vi "DeleteLongFolderStuctureFromSaveAsPrevious.vi"(8 "error in (no error)":errorcluster, 11 "Path":path) -> ()   [LabVIEW 2016]
panel:
  out "appended path":path
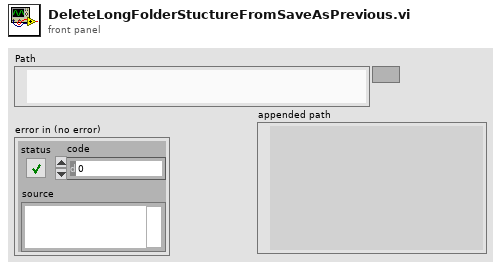
[diagram p1: front panel]
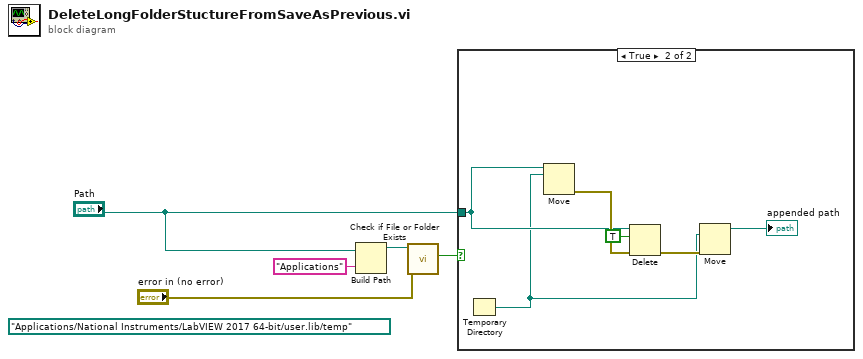
[diagram p0: block diagram]
diagram:
  (unwired) path "Applications/National Instruments/LabVIEW 2017 64-bit/user.lib/temp" ("Path")
  n1 = Build Path(base path="Path", name or relative path="Applications") -> (appended path=w1:path)
  n2 = call <vilib>:"Check if File or Folder Exists.vi"("error in (no error)"="error in (no error)", "path"=w1) -> ("file or folder exists?"=w3:bool)  [unwired: 7 in, 2 out]
  n3 = case shown="True" w3 {
    tunnel: "Path" -> [_ w7]
    frame False {
    }
    frame True {
      n4 = Temporary Directory() -> (w6:path)
      n5 = Move(source path=w7, 10:w6) -> (error out=w11:errorcluster)  [unwired: 3 in, 2 out]
      n6 = Delete(path (use dialog)=w7, entire hierarchy (F)=TRUE, error in=w11) -> (error out=w9:errorcluster)  [unwired: 2 in, 2 out]
      n7 = Move(error in=w9, 10:w6) -> (3:→"appended path":path)  [unwired: 3 in, 2 out]
    }
  }
